vi "Read state.vi"(11 "Experiment in":refnum<class "Experiment.lvclass">) -> (2 "state":T1(ring), 3 "Experiment out":refnum<class "Experiment.lvclass">)   [LabVIEW 2013, in "Experiment.lvclass"]
uses:
  Experiment.lvclass
  Experiment.lvclass/Experiment.ctl
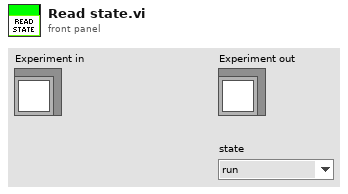
[diagram p1: front panel]
types:
  T1 = enum16{"run", "pause", "shutdown gracefully", "halt immediately"}
  T2 = typedef "states.ctl" = enum16{"run", "pause", "shutdown gracefully", "halt immediately", "waiting for connection", "waiting for command"}
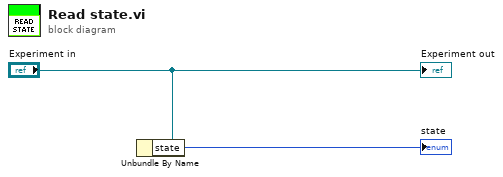
[diagram p0: block diagram]
diagram:
  n1 = Unbundle By Name("Experiment in") -> ("state"=→"state":T2)
  "Experiment out" <- "Experiment in"
